vi "phase_maps_to_pixel_difference_float_new2.vi"(10 "dist phase map":dbl[][](array[numeric]), 11 "oirg phase map":dbl[][](array[numeric])) -> (2 "displacement map 2":dbl[][](array[numeric]), 3 "displacement map":i32[][](array[numeric]))   [LabVIEW 2011]
doc: "The input array must be unwrapped phase maps, that are normalize to the same span (i.e. 0 to 255) and where the masked pixels are 0."
uses:
  global_vars.vi
panel:
  out "input":dbl[][](graph)
  in  "dbl_pxar_orig_unwrap":dbl[][](array[numeric])=array1050x1050[1102500 elements]
  in  "dbl_pxar_dist_unwrap":dbl[][](array[numeric])=array1050x1050[1102500 elements]
  in  "Stop":bool
  out "displacement":i32[](graph)
  in  "row":i32(slide) scale=0.0..1000.0
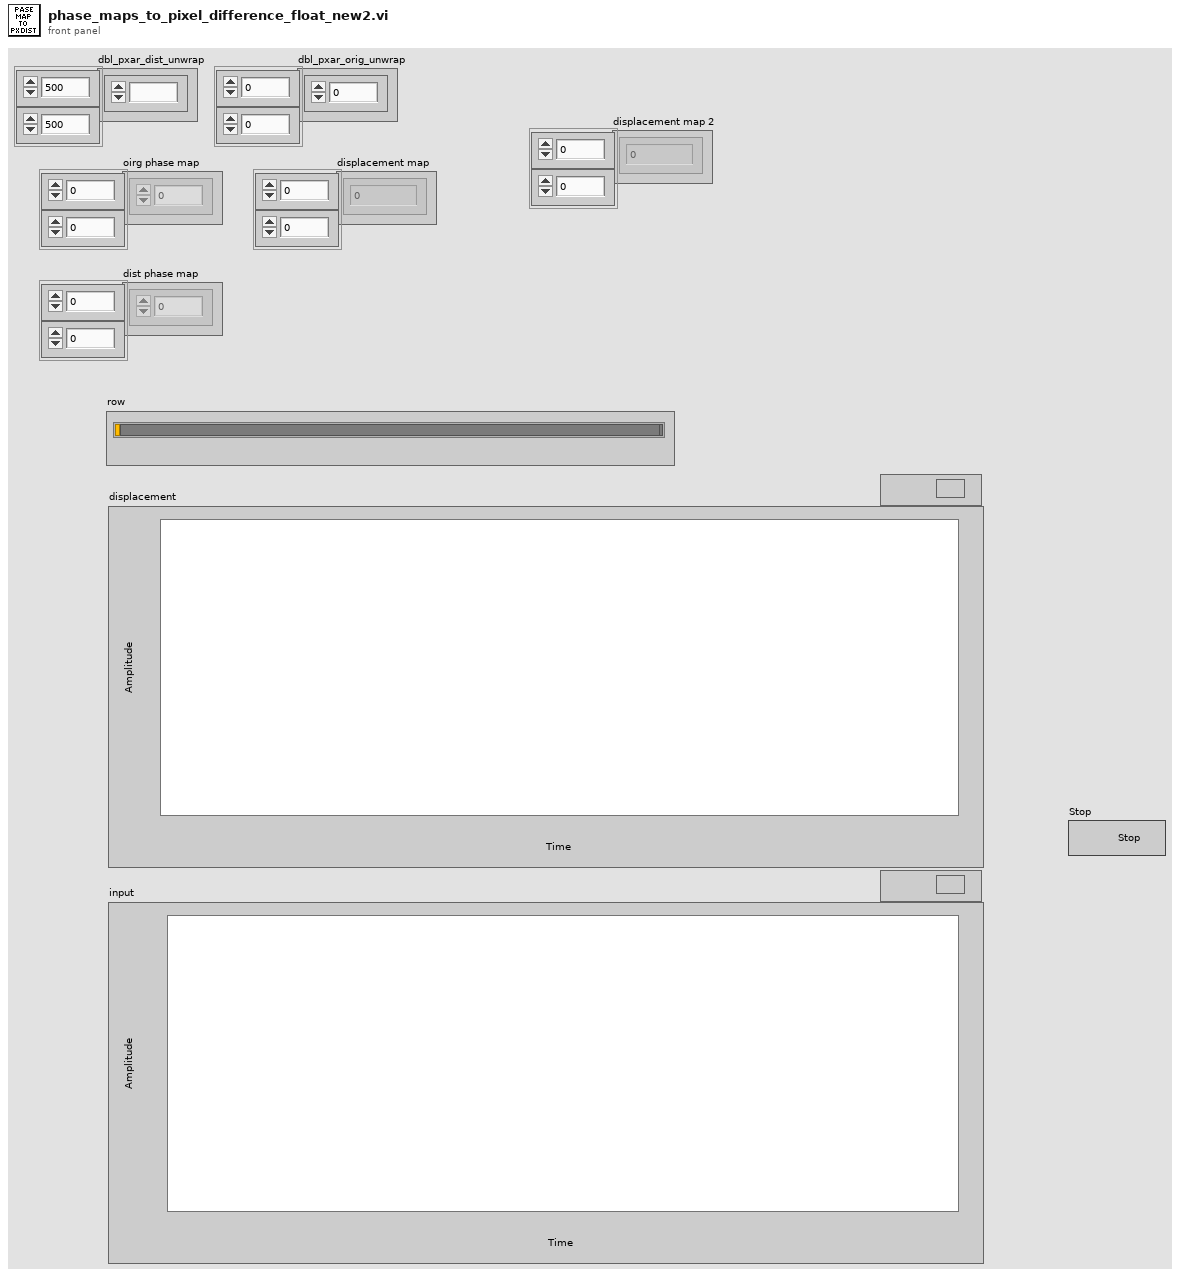
[diagram p1: front panel]
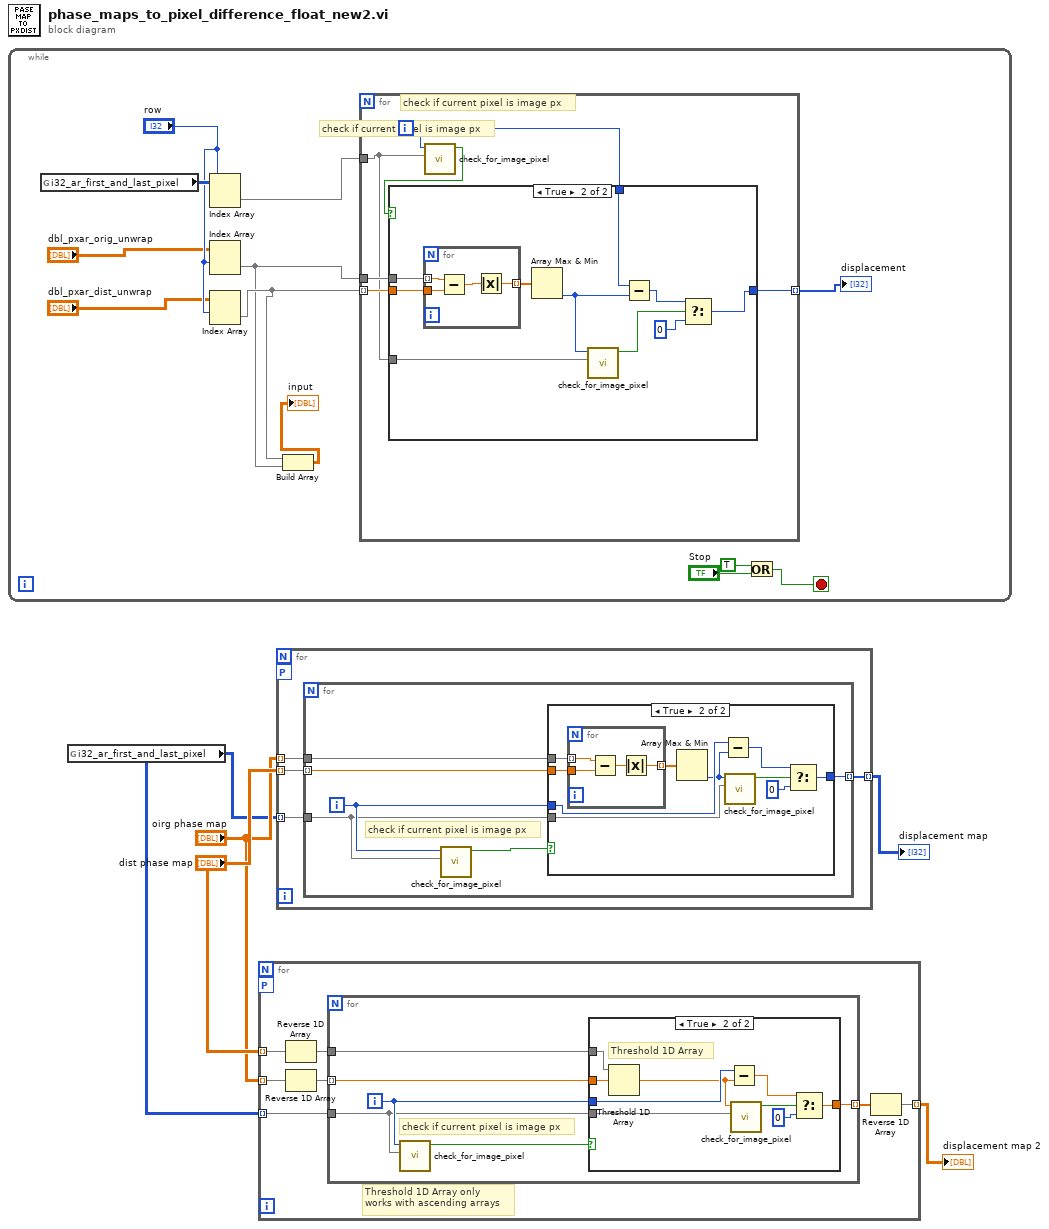
[diagram p0: block diagram]
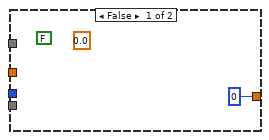
[diagram p2: hidden frame]
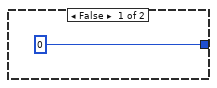
[diagram p3: hidden frame]
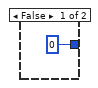
[diagram p4: hidden frame]
diagram:
  n1 = while {
    stop <- w14 stop-if-true
    # "check if current pixel is image px"
    n2 = global read "global_vars.vi" "i32_ar_first_and_last_pixel"() -> (w17:i32[][])
    n3 = Index Array(array=w17, index (row)="row") -> (element=w15:i32[])  [unwired: 1 in]
    n4 = Index Array(array="dbl_pxar_orig_unwrap", index (row)="row") -> (element=w7:dbl[])  [unwired: 1 in]
    n5 = Index Array(array="dbl_pxar_dist_unwrap", index (row)="row") -> (element=w8:dbl[])  [unwired: 1 in]
    n6 = Build Array(w8, w7) -> (→"input":dbl[][])
    n7 = for {
      tunnel: w8 -> [w23] mode=indexing
      tunnel: [w22] -> w9 mode=indexing
      tunnel: w7 -> [w21]
      tunnel: w15 -> [w18]
      i -> [w19]
      # "check if current pixel is image px"
      n8 = call "check_for_image_pixel.vi"("i32_ar_first_and_last_pixel"=w18, "current index"=w19) -> ("image pixel"=w20:bool)  [unwired: 9 in]
      n9 = case shown="True" w20 {
        tunnel: w23 -> [_ w34]
        tunnel: [0 w29] -> w22
        tunnel: w21 -> [_ w32]
        tunnel: w19 -> [_ w31]
        tunnel: w18 -> [_ w28]
        frame False {
        }
        frame True {
          n10 = for {
            tunnel: w32 -> [w38] mode=indexing
            tunnel: w34 -> [w37]
            tunnel: [w36] -> w33 mode=indexing
            n11 = Subtract(x=w38, y=w37) -> (x-y=w35:dbl)
            n12 = Absolute Value(x=w35) -> (abs(x)=w36:dbl)
          }
          n13 = Array Max & Min(array=w33) -> (min index (indices)=w27:i32)  [unwired: 3 out]
          n14 = call "check_for_image_pixel.vi"("i32_ar_first_and_last_pixel"=w28, "current index"=w27) -> ("image pixel"=w26:bool)  [unwired: 9 in]
          n15 = Subtract(x=w31, y=w27) -> (x-y=w30:i32)
          n16 = Select(t=w30, s=w26, f=0) -> (s? t:f=w29:i32)
        }
      }
    }
    "displacement" <- w9
    n17 = Or(x=TRUE, y="Stop") -> (x .or. y?=w14:bool)
  }
  n18 = global read "global_vars.vi" "i32_ar_first_and_last_pixel"() -> (w2:i32[][])
  n19 = for {
    tunnel: "dist phase map" -> [w43] mode=indexing
    tunnel: "oirg phase map" -> [w42] mode=indexing
    workers-P: _ -> [_]
    tunnel: [w39] -> w1 mode=indexing
    tunnel: w2 -> [w41] mode=indexing
    # "Threshold 1D Array only\nworks with ascending arrays"
    n20 = Reverse 1D Array(array=w43) -> (reversed array=w45:dbl[])
    n21 = Reverse 1D Array(array=w42) -> (reversed array=w44:dbl[])
    n22 = for {
      tunnel: w45 -> [w51]
      tunnel: [w50] -> w40 mode=indexing
      tunnel: w44 -> [w49] mode=indexing
      tunnel: w41 -> [w46]
      i -> [w47]
      # "check if current pixel is image px"
      n23 = call "check_for_image_pixel.vi"("i32_ar_first_and_last_pixel"=w46, "current index"=w47) -> ("image pixel"=w48:bool)  [unwired: 9 in]
      n24 = case shown="True" w48 {
        tunnel: w51 -> [_ w58]
        tunnel: [0 w61] -> w50
        tunnel: w49 -> [_ w57]
        tunnel: w47 -> [_ w56]
        tunnel: w46 -> [_ w53]
        frame False {
          (unwired) FALSE ("image pixel")
          (unwired) 0.0
        }
        frame True {
          # "Threshold 1D Array"
          n25 = Threshold 1D Array(2:w57, 3:w58) -> (0:w55:dbl)  [unwired: 1 in]
          n26 = Subtract(x=w56, y=w55) -> (x-y=w59:dbl)
          n27 = call "check_for_image_pixel.vi"("i32_ar_first_and_last_pixel"=w53, "current index"=w55) -> ("image pixel"=w54:bool)  [unwired: 9 in]
          n28 = Select(t=w59, s=w54, f=0) -> (s? t:f=w61:dbl)
        }
      }
    }
    n29 = Reverse 1D Array(array=w40) -> (reversed array=w39:dbl[])
  }
  "displacement map 2" <- w1
  n30 = for {
    tunnel: "dist phase map" -> [w65] mode=indexing
    tunnel: "oirg phase map" -> [w64] mode=indexing
    workers-P: _ -> [_]
    tunnel: [w63] -> w5 mode=indexing
    tunnel: w2 -> [w62] mode=indexing
    n31 = for {
      tunnel: w65 -> [w71] mode=indexing
      tunnel: [w70] -> w63 mode=indexing
      tunnel: w64 -> [w69]
      tunnel: w62 -> [w66]
      i -> [w67]
      # "check if current pixel is image px"
      n32 = call "check_for_image_pixel.vi"("i32_ar_first_and_last_pixel"=w66, "current index"=w67) -> ("image pixel"=w68:bool)  [unwired: 9 in]
      n33 = case shown="True" w68 {
        tunnel: w71 -> [_ w82]
        tunnel: [0 w77] -> w70
        tunnel: w69 -> [_ w80]
        tunnel: w67 -> [_ w79]
        tunnel: w66 -> [_ w76]
        frame False {
        }
        frame True {
          n34 = for {
            tunnel: w80 -> [w86] mode=indexing
            tunnel: w82 -> [w85]
            tunnel: [w84] -> w81 mode=indexing
            n35 = Subtract(x=w86, y=w85) -> (x-y=w83:dbl)
            n36 = Absolute Value(x=w83) -> (abs(x)=w84:dbl)
          }
          n37 = Array Max & Min(array=w81) -> (min index (indices)=w75:i32)  [unwired: 3 out]
          n38 = Subtract(x=w79, y=w75) -> (x-y=w78:i32)
          n39 = call "check_for_image_pixel.vi"("i32_ar_first_and_last_pixel"=w76, "current index"=w75) -> ("image pixel"=w74:bool)  [unwired: 9 in]
          n40 = Select(t=w78, s=w74, f=0) -> (s? t:f=w77:i32)
        }
      }
    }
  }
  "displacement map" <- w5
